vi "auto_serenity.vi"() -> ()   [LabVIEW 2012, in "BlockParty4150.lvrbt"]
uses:
  BlockParty4150.lvrbt
  <vilib>/NXT/Subs/LVHSConnector.ctl
  <vilib>/NXT/LegoClasses/BrickReference/BrickReference.lvclass
  <vilib>/NXT/Block Support/NXT_ButtonSelector.ctl
  <vilib>/NXT/HiTechnic/HiTechnic Controls/HiTechnic Port.ctl
  <vilib>/NXT/Block Support/NXT_InputPort.ctl
  <vilib>/NXT/Hardware/Plugins/Tetrix 180 deg Servo/Tetrix180ServoAddress.ctl
  <vilib>/NXT/Hardware/Plugins/Tetrix DC Motor/TetrixDCMotorAddress.ctl
  <vilib>/NXT/Dual Mode Library/Display/drawText.vi
  <vilib>/NXT/Dual Mode Library/Sound/Tone.vi
  <vilib>/NXT/NXTIO Xnodes/NXTIONodeSubVIs/TETRIX IO Move Servos.vi
  <vilib>/NXT/Dual Mode Library/Waits/Wait_Num(msec).vi
  <vilib>/NXT/Dual Mode Library/prims/inRangeAndCoerce/inRangeAndCoerce_int.vi
  <vilib>/NXT/Dual Mode Library/Display/drawNumber.vi
  <vilib>/NXT/NXTIO Xnodes/NXTIONodeSubVIs/TETRIX IO Move DC Motors.vi
  <vilib>/NXT/NXTIO Xnodes/NXTIONodeSubVIs/TETRIX IO Stop DC Motors.vi
  <vilib>/NXT/NXTIO Xnodes/AddressXNode/NXTIOAddress.xnode
  <vilib>/NXT/NXTIO Xnodes/NXTIOXNode/NXTIO.xnode
panel:
  out "Enabled":bool
  out "iter":i32
  out "NXT":T1
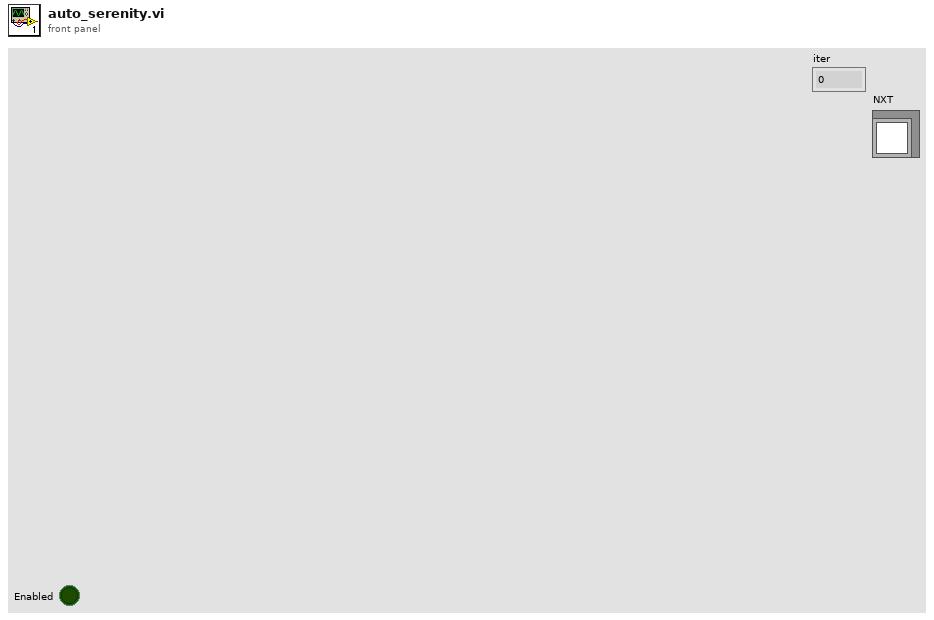
[diagram p1: front panel]
types:
  T1 = typedef "LVHSConnector.ctl" = refnum<class "BrickReference.lvclass">
  T2 = typedef "NXT_ButtonSelector.ctl" = u16
  T3 = typedef "Tetrix180ServoAddress.ctl" = i16
  T4 = typedef "TetrixDCMotorAddress.ctl" = i16
  T5 = typedef "HiTechnic Port.ctl" = cluster{"Port":T6, "MUX Port":u8}
  T6 = typedef "NXT_InputPort.ctl" = u8
  T7 = cluster{"Direction (0-9)":i16, "Signal Strength (Array)":u8[]}
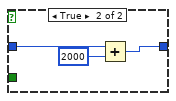
[diagram p4: hidden frame]
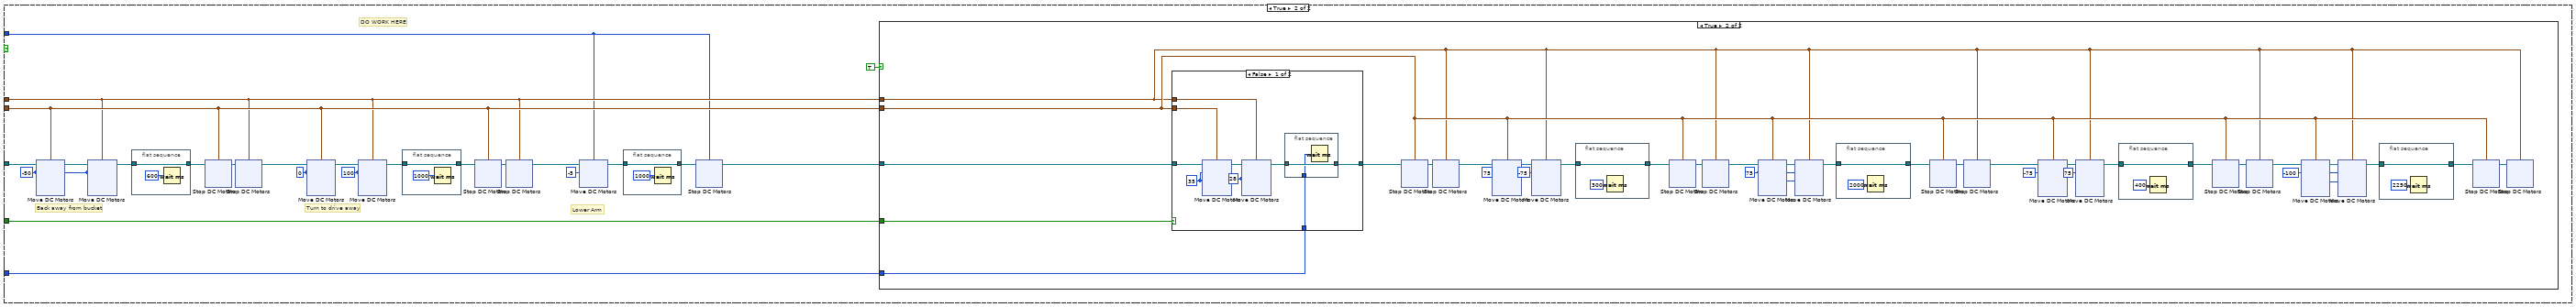
[diagram p6: hidden frame]
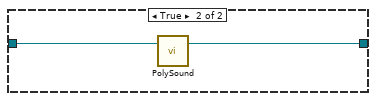
[diagram p8: hidden frame]
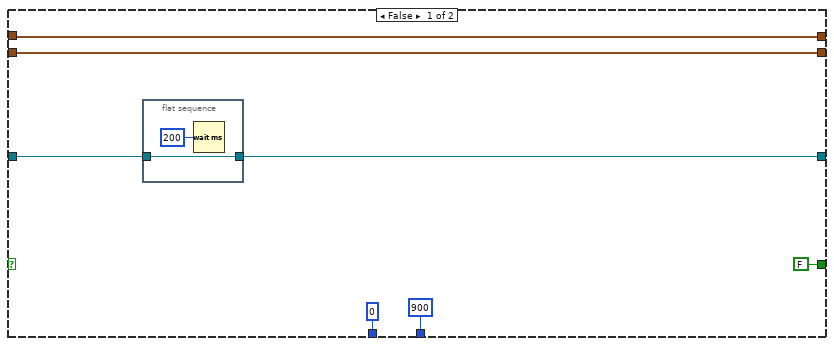
[diagram p10: hidden frame]
diagram:
  w7 = i16 4 items=["1", "2", "3", "4", "5", "6", "7", "8"] ("Line")
  w8 = i16 4 items=["1", "2", "3", "4", "5", "6", "7", "8"] ("Line")
  w14 = i8 -75 ("Power/Speed 1")
  w48 = i8 -75 ("Power/Speed 1")
  w49 = i8 0 ("Power/Speed 1")
  # "Drive back"
  # "Turn to line up"
  # "Sweep Blocks"
  n1 = local read "NXT"() -> (w1:T1)
  n2 = while {
    tunnel: [w75] -> w10
    tunnel: w1 -> [w75]
    shift-right: [w68] -> w11
    shift-left: u32 0 ("Power/Speed 1") -> [w61]
    stop <- w73 stop-if-true
    w67 = i16 2 items=["1", "2", "3", "4", "5", "6", "7", "8"] ("Line")
    w70 = T2 1 items=["Enter button"=3, "Left button"=2, "Right button"=1] ("Button (Enter button)")
    w69 = T2 2 items=["Enter button"=3, "Left button"=2, "Right button"=1] ("Button (Enter button)")
    w74 = T2 3 items=["Enter button"=3, "Left button"=2, "Right button"=1] ("Button (Enter button)")
    n3 = call-poly <vilib>:"inRangeAndCoerce_poly.vi"("lower limit"=0, "x"=w61, "upper limit"=20000) -> ("In Range?"=w56:bool, "coerced(x)"=w58:i32)
    n4 = To Unsigned Long Integer(number=w58) -> (unsigned 32bit integer=w57:u32)
    n5 = flat-sequence {
      frame #0 {
        n6 = Wait (ms)(milliseconds to wait=u32 250) -> ()  [unwired: 1 out]
      }
    }
    n7 = case shown="False" w56 {
      frame False {
        n8 = call-poly <vilib>:"PolySound.vi"("Tone (440 Hz)"=u16 220) -> ()  [unwired: 3 in, 1 out]
      }
      frame True {
      }
    }
    n9 = To Double Precision Float(number=u32 1000 ("Power/Speed 1")) -> (double precision float=w62:dbl)
    n10 = To Double Precision Float(number=w57) -> (double precision float=w64:dbl)
    n11 = Divide(x=w64, y=w62) -> (x/y=w65:dbl)
    n12 = To Long Integer(number=w65) -> (32bit integer=w63:i32)
    n13 = call-poly <vilib>:"PolyDisplay.vi"("number"=w63, "Line"=w67) -> ()  [unwired: 2 in, 1 out]
    n14 = call <vilib>:"readNXTButton.vi"("Button (Enter button)"=w69) -> ("Yes/No"=w72:bool)  [unwired: 2 in, 1 out]
    n15 = call <vilib>:"readNXTButton.vi"("Button (Enter button)"=w70) -> ("Yes/No"=w71:bool)  [unwired: 2 in, 1 out]
    n16 = case shown="False" w71 {
      tunnel: w72 -> [w80 _]
      tunnel: [w79 w86] -> w68
      tunnel: w57 -> [w78 w87]
      frame False {
        n17 = case shown="True" w80 {
          tunnel: [w81 w83] -> w79
          tunnel: w78 -> [w81 w84]
          frame False {
          }
          frame True {
            n18 = Subtract(x=w84, y=u32 2000) -> (x-y=w83:u32)
          }
        }
      }
      frame True {
        n19 = Add(x=w87, y=u32 2000) -> (x+y=w86:u32)
      }
    }
    n20 = call-poly <vilib>:"PolySensor.vi"("Button (Enter button)"=w74) -> ("Yes/No"=w73:bool)  [unwired: 2 in, 1 out]
  }
  n21 = call-poly <vilib>:"PolyDisplay.vi"("Text"="Wait Entered!", "NXT"=w10, "Line"=w8) -> ("NXT"=w3:T1)  [unwired: 1 in]
  n22 = while {
    tunnel: [w88] -> w2
    tunnel: w3 -> [w88]
    stop <- w89 stop-if-true
    n23 = local read "Enabled"() -> (w89:bool)
  }
  n24 = call-poly <vilib>:"PolyDisplay.vi"("Text"="Counting down", "NXT"=w2, "Line"=w7) -> ("NXT"=w5:T1)  [unwired: 1 in]
  n25 = flat-sequence {
    tunnel: w5 -> [w91]
    tunnel: [w91] -> w13
    tunnel: w11 -> [w90]
    frame #0 {
      n26 = Wait (ms)(milliseconds to wait=w90) -> ()  [unwired: 1 out]
    }
  }
  n27 = xnode "Motors"() -> ("Motor"=w31:T3)
  n28 = call-poly <vilib>:"PolySound.vi"("NXT"=w13) -> ("NXT"=w4:T1)  [unwired: 3 in]
  n29 = xnode "Motors"() -> ("Motor"=w30:cluster{"TetrixDCMotor":T4, "TetrixDCMotor":T4})
  n30 = xnode "Motors"() -> ("Motor"=w32:T4)
  n31 = xnode "Motors"() -> ("Motor"=w15:cluster{"TetrixDCMotor":T4, "TetrixDCMotor":T4})
  n32 = xnode "Move Servos"("Position 1"=u8 75, "Servos"=w31) -> ("NXT"=w54:T1)  [unwired: 1 in]
  n33 = xnode "Move DC Motors"("Power/Speed 1"=i8 100, "Motors"=w32, "NXT"=w4) -> ("NXT"=w52:T1)
  n34 = while {
    tunnel: w54 -> [_]
    i -> [w93]
    stop <- FALSE stop-if-true
    # "Communicates with the FCS and enables \nor disables the robot as neccessary."
    n35 = call <vilib>:"FTC Read Latest Packet.vi"() -> ("Packet Received?"=w103:bool, "Stopped?"=w102:bool, "NXT"=w105:T1)  [unwired: 6 in, 3 out]
    n36 = call <vilib>:"FTC Get Connection Status.vi"("Packet Received?"=w103, "Stopped?"=w102, "NXT"=w105) -> ("Online?"=w95:bool, "Stopped?"=w96:bool, "NXT"=w104:T1)  [unwired: 5 in]
    n37 = call <vilib>:"FTC Disable Robot.vi"("Online?"=w95, "Stopped?"=w96, "NXT"=w104) -> ("Enabled?"=w99:enum16{"Disabled", "Enabled"}, "NXT"=w101:T1)  [unwired: 3 in]
    n38 = Equal?(x=w99, y=enum16{"Disabled", "Enabled"}."Enabled") -> (x = y?=→"Enabled":bool)
    n39 = call-poly <vilib>:"PolyWait.vi"("Time (100 msec)"=u32 50 ("Time (msec)"), "NXT"=w101) -> ("NXT"=→"NXT":T1)  [unwired: 2 in]
    "iter" <- w93
  }
  n40 = flat-sequence {
    tunnel: w52 -> [w106]
    tunnel: [w106] -> w51
    frame #0 {
      n41 = Wait (ms)(milliseconds to wait=u32 3000) -> ()  [unwired: 1 out]
    }
  }
  n42 = xnode "Stop DC Motors"("Motors"=w32, "NXT"=w51) -> ("NXT"=w39:T1)
  n43 = xnode "Move DC Motors"("Power/Speed 2"=w14, "Power/Speed 1"=w14, "Motors"=w15, "NXT"=w39) -> ("NXT"=w40:T1)
  n44 = xnode "Move DC Motors"("Power/Speed 2"=w14, "Power/Speed 1"=w14, "Motors"=w30, "NXT"=w40) -> ("NXT"=w42:T1)
  n45 = flat-sequence {
    tunnel: w42 -> [w108]
    tunnel: [w108] -> w41
    frame #0 {
      n46 = Wait (ms)(milliseconds to wait=u32 550) -> ()  [unwired: 1 out]
    }
  }
  n47 = xnode "Stop DC Motors"("Motors"=w15, "NXT"=w41) -> ("NXT"=w43:T1)
  n48 = xnode "Stop DC Motors"("Motors"=w30, "NXT"=w43) -> ("NXT"=w38:T1)
  n49 = xnode "Move DC Motors"("Power/Speed 2"=w49, "Power/Speed 1"=w49, "Motors"=w15, "NXT"=w38) -> ("NXT"=w50:T1)
  n50 = xnode "Move DC Motors"("Power/Speed 2"=w48, "Power/Speed 1"=w48, "Motors"=w30, "NXT"=w50) -> ("NXT"=w46:T1)
  n51 = flat-sequence {
    tunnel: w46 -> [w110]
    tunnel: [w110] -> w47
    frame #0 {
      n52 = Wait (ms)(milliseconds to wait=u32 800) -> ()  [unwired: 1 out]
    }
  }
  n53 = xnode "Stop DC Motors"("Motors"=w15, "NXT"=w47) -> ("NXT"=w45:T1)
  n54 = xnode "Stop DC Motors"("Motors"=w30, "NXT"=w45) -> ("NXT"=w44:T1)
  n55 = flat-sequence {
    tunnel: w44 -> [w113]
    tunnel: [w113] -> w36
    frame #0 {
      n56 = Wait (ms)(milliseconds to wait=u32 0) -> ()  [unwired: 1 out]
    }
  }
  n57 = flat-sequence {
    tunnel: [w114] -> w37
    tunnel: w36 -> [_]
    frame #0 {
      n58 = Tick Count (ms)() -> (millisecond timer value=w114:u32)
    }
  }
  n59 = while {
    tunnel: w36 -> [w129]
    tunnel: w37 -> [w136]
    tunnel: [w135] -> w17
    tunnel: [w131] -> w33
    tunnel: w15 -> [w127]
    tunnel: w30 -> [w126]
    tunnel: [w118] -> w34
    tunnel: [w117] -> w35
    stop <- w134 stop-if-true
    w115 = i8 28 ("Power/Speed 2")
    w116 = i8 35 ("Power/Speed 1")
    w117 = u32 1500 ("y")
    n60 = xnode "Move DC Motors"("Power/Speed 2"=w116, "Power/Speed 1"=w116, "Motors"=w127, "NXT"=w129) -> ("NXT"=w130:T1)
    n61 = xnode "Move DC Motors"("Power/Speed 2"=w115, "Power/Speed 1"=w115, "Motors"=w126, "NXT"=w130) -> ("NXT"=w128:T1)
    n62 = Tick Count (ms)() -> (millisecond timer value=w137:u32)
    n63 = call <vilib>:"HiTechnic IRSeeker Sensor_AC all.vi"("NXT"=w128, "Port/MUX"=T5 {"Port"=3, "MUX Port"=0}) -> ("All Info"=w139:T7, "NXT"=w135:T1)  [unwired: 1 in]
    n64 = Subtract(x=w137, y=w136) -> (x-y=w118:u32)
    n65 = Unbundle By Name(w139) -> ("Direction (0-9)"=w132:i16, "Signal Strength (Array)"=w125:u8[])
    n66 = Greater Or Equal?(x=w118, y=w117) -> (x >= y?=w131:bool)
    n67 = Index Array(array=w125, index=3) -> (element=w123:u8)
    n68 = Less Or Equal?(x=w123, y=u8 50) -> (x <= y?=w120:bool)
    n69 = Greater Or Equal?(x=w132, y=i16 7 ("Direction")) -> (x >= y?=w121:bool)
    n70 = And(x=w121, y=w120) -> (x .and. y?=w119:bool)
    n71 = Or(x=w119, y=w131) -> (x .or. y?=w134:bool)
    n72 = call <vilib>:"FeedAllTETRIXWatchdogs.vi"() -> ()  [unwired: 11 in, 1 out]
  }
  n73 = case shown="True" w33 {
    tunnel: [w163 w176] -> w29
    tunnel: w30 -> [w161 w170]
    tunnel: w15 -> [w160 w169]
    tunnel: w17 -> [w162 w174]
    tunnel: [FALSE w173] -> w23
    tunnel: [u32 900 ("y") w172] -> w28
    tunnel: [u32 0 w171] -> w26
    tunnel: [w161 w170] -> w18
    tunnel: [w160 w169] -> w19
    frame False {
      n74 = flat-sequence {
        tunnel: [w167] -> w163
        tunnel: w162 -> [w167]
        frame #0 {
          n75 = Wait (ms)(milliseconds to wait=u32 200) -> ()  [unwired: 1 out]
        }
      }
    }
    frame True {
      n76 = flat-sequence {
        tunnel: [w177] -> w175
        tunnel: w174 -> [_]
        frame #0 {
          n77 = Tick Count (ms)() -> (millisecond timer value=w177:u32)
        }
      }
      n78 = while {
        tunnel: w174 -> [w178]
        tunnel: w175 -> [w193]
        tunnel: [w192] -> w176
        tunnel: [w188] -> w173
        tunnel: [w180] -> w171
        tunnel: [w179] -> w172
        stop <- w191 stop-if-true
        w179 = u32 900 ("y")
        n79 = Tick Count (ms)() -> (millisecond timer value=w194:u32)
        n80 = call <vilib>:"HiTechnic IRSeeker Sensor_AC all.vi"("NXT"=w178, "Port/MUX"=T5 {"Port"=3, "MUX Port"=0}) -> ("All Info"=w196:T7, "NXT"=w192:T1)  [unwired: 1 in]
        n81 = Subtract(x=w194, y=w193) -> (x-y=w180:u32)
        n82 = Unbundle By Name(w196) -> ("Direction (0-9)"=w189:i16, "Signal Strength (Array)"=w187:u8[])
        n83 = Greater Or Equal?(x=w180, y=w179) -> (x >= y?=w188:bool)
        n84 = Index Array(array=w187, index=3) -> (element=w185:u8)
        n85 = Less Or Equal?(x=w185, y=u8 47) -> (x <= y?=w182:bool)
        n86 = Greater Or Equal?(x=w189, y=i16 6 ("Direction")) -> (x >= y?=w183:bool)
        n87 = And(x=w183, y=w182) -> (x .and. y?=w181:bool)
        n88 = Or(x=w181, y=w188) -> (x .or. y?=w191:bool)
        n89 = call <vilib>:"FeedAllTETRIXWatchdogs.vi"() -> ()  [unwired: 11 in, 1 out]
      }
    }
  }
  n90 = Add(x=w28, y=w35) -> (x+y=w27:u32)
  n91 = Add(x=w26, y=w34) -> (x+y=w25:u32)
  n92 = Subtract(x=w27, y=w25) -> (x-y=w24:u32)
  n93 = flat-sequence {
    tunnel: [w197] -> w21
    tunnel: w29 -> [w197]
    frame #0 {
      n94 = Wait (ms)(milliseconds to wait=u32 150) -> ()  [unwired: 1 out]
    }
  }
  n95 = xnode "Stop DC Motors"("Motors"=w19, "NXT"=w21) -> ("NXT"=w22:T1)
  n96 = xnode "Stop DC Motors"("Motors"=w18, "NXT"=w22) -> ("NXT"=w20:T1)
  n97 = case shown="True" TRUE {
    tunnel: w32 -> [_ w229]
    tunnel: w24 -> [_ w228]
    tunnel: w23 -> [_ w227]
    tunnel: w20 -> [_ w220]
    tunnel: w19 -> [_ w203]
    tunnel: w18 -> [_ w202]
    frame False {
    }
    frame True {
      w212 = i8 50 ("Power/Speed 1")
      w223 = i8 -100 ("Power/Speed 1")
      w222 = i8 0 ("Power/Speed 1")
      # "Raise Arm"
      # "Approach bucket"
      # "Spit block out"
      # "Back Up to bucket"
      n98 = xnode "Move DC Motors"("Power/Speed 2"=w222, "Power/Speed 1"=w222, "Motors"=w203, "NXT"=w220) -> ("NXT"=w221:T1)
      n99 = xnode "Move DC Motors"("Power/Speed 2"=w223, "Power/Speed 1"=w223, "Motors"=w202, "NXT"=w221) -> ("NXT"=w225:T1)
      n100 = flat-sequence {
        tunnel: w225 -> [w708]
        tunnel: [w708] -> w224
        frame #0 {
          n101 = Wait (ms)(milliseconds to wait=u32 1100) -> ()  [unwired: 1 out]
        }
      }
      n102 = xnode "Stop DC Motors"("Motors"=w203, "NXT"=w224) -> ("NXT"=w226:T1)
      n103 = xnode "Stop DC Motors"("Motors"=w202, "NXT"=w226) -> ("NXT"=w207:T1)
      n104 = xnode "Motors"() -> ("Motor"=w201:T4)
      n105 = xnode "Move DC Motors"("Power/Speed 1"=i8 60, "Motors"=w201, "NXT"=w207) -> ("NXT"=w210:T1)
      n106 = flat-sequence {
        tunnel: w210 -> [w634]
        tunnel: [w634] -> w211
        frame #0 {
          n107 = Wait (ms)(milliseconds to wait=u32 1000) -> ()  [unwired: 1 out]
        }
      }
      n108 = xnode "Stop DC Motors"("Motors"=w201, "NXT"=w211) -> ("NXT"=w208:T1)
      n109 = xnode "Move DC Motors"("Power/Speed 2"=w212, "Power/Speed 1"=w212, "Motors"=w203, "NXT"=w208) -> ("NXT"=w216:T1)
      n110 = xnode "Move DC Motors"("Power/Speed 2"=w212, "Power/Speed 1"=w212, "Motors"=w202, "NXT"=w216) -> ("NXT"=w214:T1)
      n111 = flat-sequence {
        tunnel: w214 -> [w657]
        tunnel: [w657] -> w215
        frame #0 {
          n112 = Wait (ms)(milliseconds to wait=u32 450) -> ()  [unwired: 1 out]
        }
      }
      n113 = xnode "Stop DC Motors"("Motors"=w203, "NXT"=w215) -> ("NXT"=w213:T1)
      n114 = xnode "Stop DC Motors"("Motors"=w202, "NXT"=w213) -> ("NXT"=w206:T1)
      n115 = case shown="True" FALSE {
        tunnel: w206 -> [w608 w611]
        tunnel: [w608 w610] -> w205
        tunnel: w201 -> [_ w609]
        frame False {
        }
        frame True {
          # "Lower Arm"
          n116 = xnode "Move DC Motors"("Power/Speed 1"=i8 -5, "Motors"=w609, "NXT"=w611) -> ("NXT"=w613:T1)
          n117 = flat-sequence {
            tunnel: w613 -> [w620]
            tunnel: [w620] -> w612
            frame #0 {
              n118 = Wait (ms)(milliseconds to wait=u32 400) -> ()  [unwired: 1 out]
            }
          }
          n119 = xnode "Stop DC Motors"("Motors"=w609, "NXT"=w612) -> ("NXT"=w610:T1)
        }
      }
      n120 = xnode "Move DC Motors"("Power/Speed 1"=i8 -40, "Motors"=w229, "NXT"=w205) -> ("NXT"=w218:T1)
      n121 = flat-sequence {
        tunnel: w218 -> [w685]
        tunnel: [w685] -> w219
        frame #0 {
          n122 = Wait (ms)(milliseconds to wait=u32 1500) -> ()  [unwired: 1 out]
        }
      }
      n123 = xnode "Stop DC Motors"("Motors"=w229, "NXT"=w219) -> ("NXT"=w204:T1)
      n124 = case shown="False" FALSE {
        tunnel: w228 -> [_ w297]
        tunnel: w227 -> [_ w296]
        tunnel: w204 -> [w232 w289]
        tunnel: w203 -> [w231 w281]
        tunnel: w202 -> [w230 w280]
        tunnel: w201 -> [_ w275]
        frame False {
          w237 = i8 -50 ("Power/Speed 1")
          # "Approach bucket"
          n125 = xnode "Move DC Motors"("Power/Speed 2"=w237, "Power/Speed 1"=w237, "Motors"=w231, "NXT"=w232) -> ("NXT"=w233:T1)
          n126 = xnode "Move DC Motors"("Power/Speed 2"=w237, "Power/Speed 1"=w237, "Motors"=w230, "NXT"=w233) -> ("NXT"=w235:T1)
          n127 = flat-sequence {
            tunnel: w235 -> [w252]
            tunnel: [w252] -> w234
            frame #0 {
              n128 = Wait (ms)(milliseconds to wait=u32 450) -> ()  [unwired: 1 out]
            }
          }
          n129 = xnode "Stop DC Motors"("Motors"=w231, "NXT"=w234) -> ("NXT"=w236:T1)
          n130 = xnode "Stop DC Motors"("Motors"=w230, "NXT"=w236) -> ()  [unwired: 1 out]
        }
        frame True {
          w286 = i8 100 ("Power/Speed 1")
          w287 = i8 0 ("Power/Speed 1")
          w294 = i8 -50 ("Power/Speed 1")
          # "Lower Arm"
          # "Turn to drive away"
          # "Back away from bucket"
          # "DO WORK HERE"
          n131 = xnode "Move DC Motors"("Power/Speed 2"=w294, "Power/Speed 1"=w294, "Motors"=w281, "NXT"=w289) -> ("NXT"=w290:T1)
          n132 = xnode "Move DC Motors"("Power/Speed 2"=w294, "Power/Speed 1"=w294, "Motors"=w280, "NXT"=w290) -> ("NXT"=w292:T1)
          n133 = flat-sequence {
            tunnel: w292 -> [w362]
            tunnel: [w362] -> w291
            frame #0 {
              n134 = Wait (ms)(milliseconds to wait=u32 600) -> ()  [unwired: 1 out]
            }
          }
          n135 = xnode "Stop DC Motors"("Motors"=w281, "NXT"=w291) -> ("NXT"=w293:T1)
          n136 = xnode "Stop DC Motors"("Motors"=w280, "NXT"=w293) -> ("NXT"=w282:T1)
          n137 = xnode "Move DC Motors"("Power/Speed 2"=w287, "Power/Speed 1"=w287, "Motors"=w281, "NXT"=w282) -> ("NXT"=w288:T1)
          n138 = xnode "Move DC Motors"("Power/Speed 2"=w286, "Power/Speed 1"=w286, "Motors"=w280, "NXT"=w288) -> ("NXT"=w284:T1)
          n139 = flat-sequence {
            tunnel: w284 -> [w326]
            tunnel: [w326] -> w285
            frame #0 {
              n140 = Wait (ms)(milliseconds to wait=u32 1000) -> ()  [unwired: 1 out]
            }
          }
          n141 = xnode "Stop DC Motors"("Motors"=w281, "NXT"=w285) -> ("NXT"=w283:T1)
          n142 = xnode "Stop DC Motors"("Motors"=w280, "NXT"=w283) -> ("NXT"=w276:T1)
          n143 = xnode "Move DC Motors"("Power/Speed 1"=i8 -5, "Motors"=w275, "NXT"=w276) -> ("NXT"=w278:T1)
          n144 = flat-sequence {
            tunnel: w278 -> [w303]
            tunnel: [w303] -> w279
            frame #0 {
              n145 = Wait (ms)(milliseconds to wait=u32 1000) -> ()  [unwired: 1 out]
            }
          }
          n146 = xnode "Stop DC Motors"("Motors"=w275, "NXT"=w279) -> ("NXT"=w274:T1)
          n147 = case shown="True" TRUE {
            tunnel: w297 -> [_ w414]
            tunnel: w296 -> [_ w413]
            tunnel: w274 -> [_ w384]
            tunnel: w281 -> [_ w386]
            tunnel: w280 -> [_ w385]
            frame False {
            }
            frame True {
              w393 = i8 -100 ("Power/Speed 1")
              w399 = i8 75 ("Power/Speed 1")
              w398 = i8 -75 ("Power/Speed 1")
              w406 = i8 75 ("Power/Speed 1")
              w412 = i8 -75 ("Power/Speed 1")
              w411 = i8 75 ("Power/Speed 1")
              n148 = case shown="False" w413 {
                tunnel: w384 -> [w568 w593]
                tunnel: w414 -> [w565 _]
                tunnel: w386 -> [w564 _]
                tunnel: w385 -> [w563 _]
                tunnel: [w561 w592] -> w415
                frame False {
                  w562 = i8 28 ("Power/Speed 2")
                  w569 = i8 35 ("Power/Speed 1")
                  n149 = xnode "Move DC Motors"("Power/Speed 2"=w569, "Power/Speed 1"=w569, "Motors"=w564, "NXT"=w568) -> ("NXT"=w567:T1)
                  n150 = xnode "Move DC Motors"("Power/Speed 2"=w562, "Power/Speed 1"=w562, "Motors"=w563, "NXT"=w567) -> ("NXT"=w566:T1)
                  n151 = flat-sequence {
                    tunnel: [w571] -> w561
                    tunnel: w566 -> [w571]
                    tunnel: w565 -> [w570]
                    frame #0 {
                      n152 = Wait (ms)(milliseconds to wait=w570) -> ()  [unwired: 1 out]
                    }
                  }
                }
                frame True {
                  n153 = call-poly <vilib>:"PolySound.vi"("NXT"=w593) -> ("NXT"=w592:T1)  [unwired: 3 in]
                }
              }
              n154 = xnode "Stop DC Motors"("Motors"=w386, "NXT"=w415) -> ("NXT"=w416:T1)
              n155 = xnode "Stop DC Motors"("Motors"=w385, "NXT"=w416) -> ("NXT"=w400:T1)
              n156 = xnode "Move DC Motors"("Power/Speed 2"=w411, "Power/Speed 1"=w411, "Motors"=w386, "NXT"=w400) -> ("NXT"=w410:T1)
              n157 = xnode "Move DC Motors"("Power/Speed 2"=w412, "Power/Speed 1"=w412, "Motors"=w385, "NXT"=w410) -> ("NXT"=w407:T1)
              n158 = flat-sequence {
                tunnel: [w539] -> w409
                tunnel: w407 -> [w539]
                frame #0 {
                  n159 = Wait (ms)(milliseconds to wait=u32 300) -> ()  [unwired: 1 out]
                }
              }
              n160 = xnode "Stop DC Motors"("Motors"=w386, "NXT"=w409) -> ("NXT"=w408:T1)
              n161 = xnode "Stop DC Motors"("Motors"=w385, "NXT"=w408) -> ("NXT"=w401:T1)
              n162 = xnode "Move DC Motors"("Power/Speed 2"=w406, "Power/Speed 1"=w406, "Motors"=w386, "NXT"=w401) -> ("NXT"=w405:T1)
              n163 = xnode "Move DC Motors"("Power/Speed 2"=w406, "Power/Speed 1"=w406, "Motors"=w385, "NXT"=w405) -> ("NXT"=w402:T1)
              n164 = flat-sequence {
                tunnel: [w503] -> w404
                tunnel: w402 -> [w503]
                frame #0 {
                  n165 = Wait (ms)(milliseconds to wait=u32 2000) -> ()  [unwired: 1 out]
                }
              }
              n166 = xnode "Stop DC Motors"("Motors"=w386, "NXT"=w404) -> ("NXT"=w403:T1)
              n167 = xnode "Stop DC Motors"("Motors"=w385, "NXT"=w403) -> ("NXT"=w387:T1)
              n168 = xnode "Move DC Motors"("Power/Speed 2"=w398, "Power/Speed 1"=w398, "Motors"=w386, "NXT"=w387) -> ("NXT"=w397:T1)
              n169 = xnode "Move DC Motors"("Power/Speed 2"=w399, "Power/Speed 1"=w399, "Motors"=w385, "NXT"=w397) -> ("NXT"=w394:T1)
              n170 = flat-sequence {
                tunnel: [w467] -> w396
                tunnel: w394 -> [w467]
                frame #0 {
                  n171 = Wait (ms)(milliseconds to wait=u32 400) -> ()  [unwired: 1 out]
                }
              }
              n172 = xnode "Stop DC Motors"("Motors"=w386, "NXT"=w396) -> ("NXT"=w395:T1)
              n173 = xnode "Stop DC Motors"("Motors"=w385, "NXT"=w395) -> ("NXT"=w388:T1)
              n174 = xnode "Move DC Motors"("Power/Speed 2"=w393, "Power/Speed 1"=w393, "Motors"=w386, "NXT"=w388) -> ("NXT"=w392:T1)
              n175 = xnode "Move DC Motors"("Power/Speed 2"=w393, "Power/Speed 1"=w393, "Motors"=w385, "NXT"=w392) -> ("NXT"=w389:T1)
              n176 = flat-sequence {
                tunnel: [w431] -> w391
                tunnel: w389 -> [w431]
                frame #0 {
                  n177 = Wait (ms)(milliseconds to wait=u32 2250) -> ()  [unwired: 1 out]
                }
              }
              n178 = xnode "Stop DC Motors"("Motors"=w386, "NXT"=w391) -> ("NXT"=w390:T1)
              n179 = xnode "Stop DC Motors"("Motors"=w385, "NXT"=w390) -> ()  [unwired: 1 out]
            }
          }
        }
      }
    }
  }
